vi "Execute Change Boolean Image Color.vi"(6 "Mouse Position":T1, 8 "User VI Ref":refnum<vi>, 9 "Menu Item Tag Suffix":string, 10 "Remaining Items":refnum<vi>[](array[refnum]), 11 "Affected Items":cluster{"Controls":refnum<vi>[]}) -> (0 "Fail transaction?":bool)   [LabVIEW 2021]
doc: "This VI will set a Boolean type that is input to the control's tag and stays persistent. It marks the data that is used in future application when changing themes.\n\n<b>Original</b>:This VI is part of a plug-in for modifying the LabVIEW shortcut menus. This is the execute VI which is called when the shortcut menu is chosen by the user. It performs the action of the selected menu item."
uses:
  Material-Scheme/Material-Scheme.lvclass
  <vilib>/Utility/miscctls.llb/LVPositionTypeDef.ctl
  Material SubVIs/Material SubVIs.lvlib
panel:
  # "All controls on this panel except \"Affected Items\" have been locked to prevent accidental edits. Changing the control names or types, other than the elements of the \"Affected Items\" cluster will make the VI unusable as a menu plugin.\n\nSee Context Help for each control for details about its use."
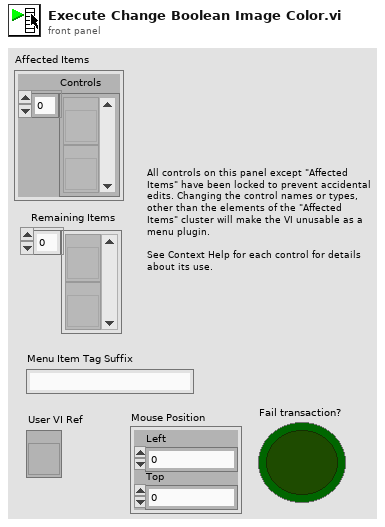
[diagram p1: front panel]
types:
  T1 = typedef "LVPositionTypeDef.ctl" = cluster{"Left":i32, "Top":i32}
  T2 = enum32{"invalid VI type", "Standard VI", "Control VI", "Global VI", "Polymorphic VI", "Configuration VI", "SubSystem", "Facade VI", "Method VI", "Statechart Diagram VI"}
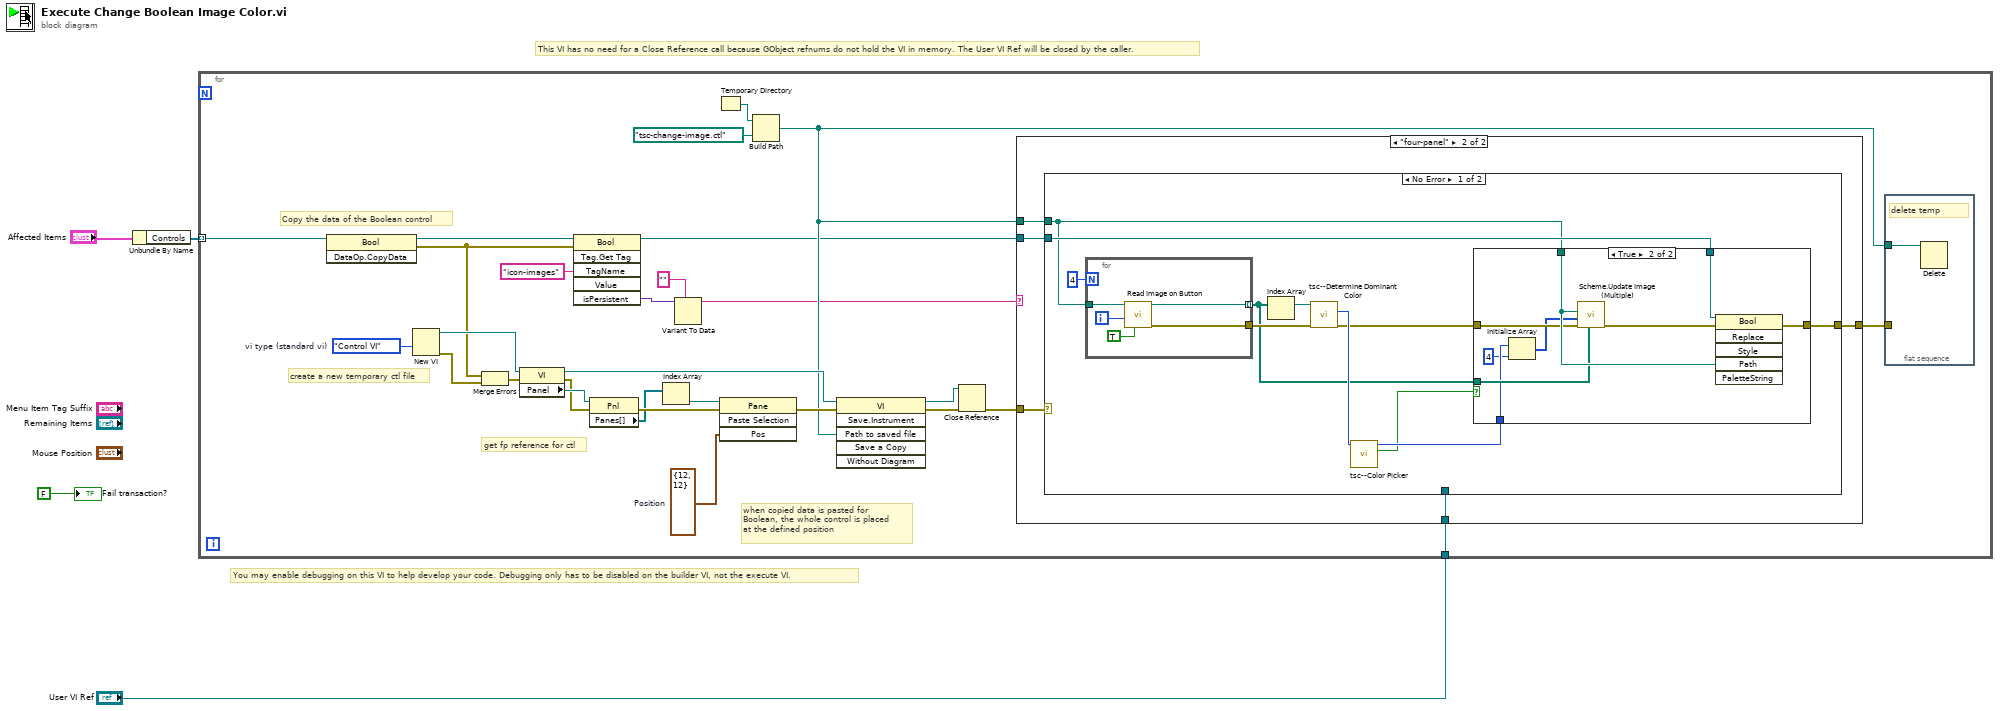
[diagram p0: block diagram]
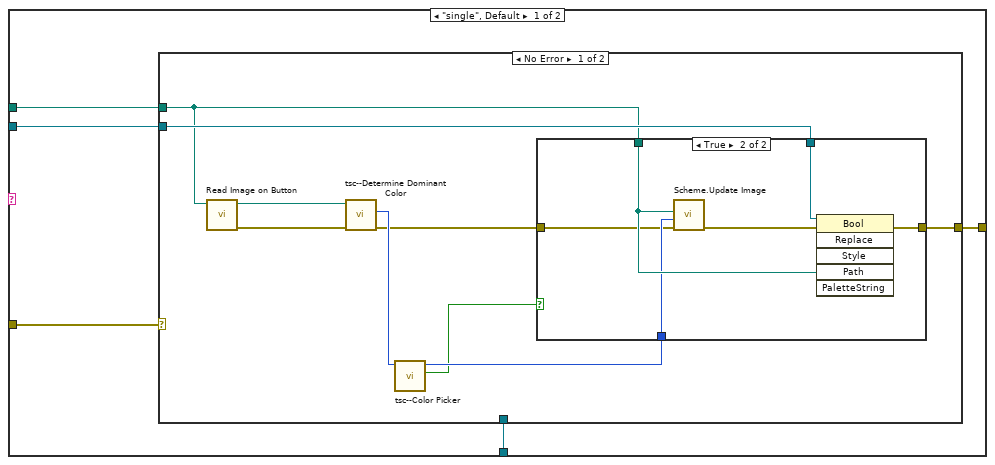
[diagram p2: hidden frame]
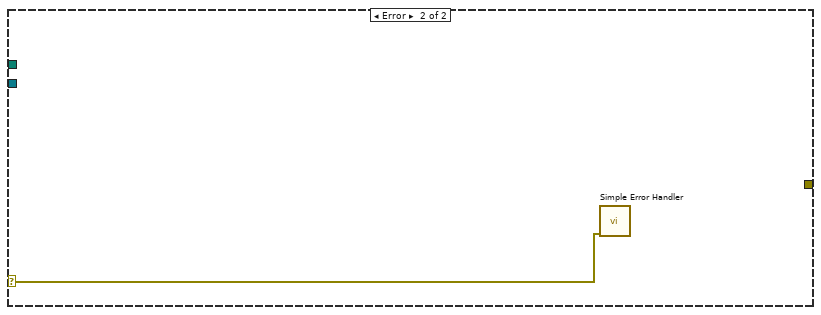
[diagram p4: hidden frame]
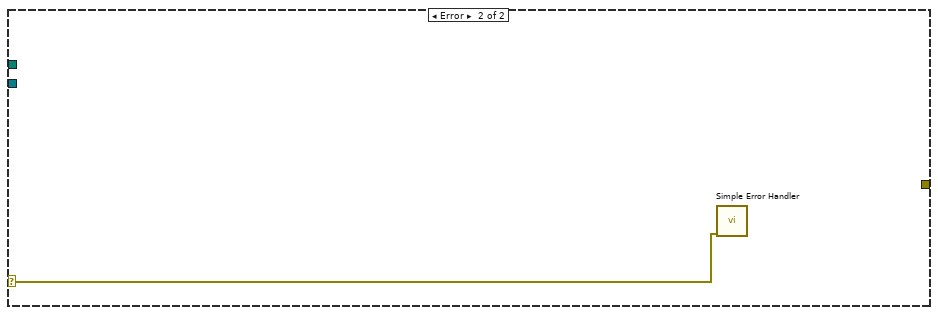
[diagram p6: hidden frame]
diagram:
  # "You may enable debugging on this VI to help develop your code. Debugging only has to be disabled on the builder VI, not the execute VI."
  # "This VI has no need for a Close Reference call because GObject refnums do not hold the VI in memory. The User VI Ref will be closed by the caller."
  n1 = Unbundle By Name("Affected Items") -> ("Controls"=w2:refnum<vi>[])
  n2 = for {
    tunnel: w2 -> [w24] mode=indexing
    tunnel: "User VI Ref" -> [w12]
    w21 = T2."Control VI"  # vi type (standard vi)
    w25 = T1 {"Left"=12, "Top"=12}  # Position
    # "when copied data is pasted for\nBoolean, the whole control is placed \nat the defined position"
    # "get fp reference for ctl"
    # "create a new temporary ctl file"
    # "Copy the data of the Boolean control"
    n3 = invoke class="Bool" method="DataOp.CopyData"(reference=w24) -> (reference out=w8:refnum<vi>, error out=w7:errorcluster)  [unwired: 2 in, 1 out]
    n4 = New VI(9:w21) -> (0:w19:errorcluster, 3:w20:refnum<vi>)  [unwired: 6 in]
    n5 = Merge Errors(w7, w19) -> (w23:errorcluster)
    n6 = property class="VI"(reference=w20, error in=w23) -> (reference out=w29:refnum<vi>, error out=w31:errorcluster, "Panel"=w32:refnum<vi>)
    n7 = invoke class="Bool" method="Tag.Get Tag"(reference=w8, error in=w7, "TagName"="icon-images" ("Tag Name")) -> (reference out=w6:refnum<vi>, "isPersistent"=w10:variant)  [unwired: 3 in, 4 out]
    n8 = property class="Pnl"(reference=w32, error in=w31) -> (error out=w28:errorcluster, "Panes[]"=w27:refnum<vi>[])  [unwired: 1 out]
    n9 = Index Array(array=w27) -> (element=w26:refnum<vi>)  [unwired: 1 in]
    n10 = Variant To Data(type="", Variant=w10) -> (data=w5:string)  [unwired: 1 in, 1 out]
    n11 = Temporary Directory() -> (w18:path)
    n12 = invoke class="Pane" method="Paste Selection"(reference=w26, error in=w28, "Pos"=w25) -> (error out=w30:errorcluster)  [unwired: 1 in, 3 out]
    n13 = Build Path(base path=w18, name or relative path=path "tsc-change-image.ctl") -> (appended path=w13:path)
    n14 = invoke class="VI" method="Save.Instrument"(reference=w29, error in=w30, "Path to saved file"=w13) -> (reference out=w15:refnum<vi>, error out=w22:errorcluster)  [unwired: 3 in, 4 out]
    n15 = Close Reference(reference=w15, error in (no error)=w22) -> (error out=w16:errorcluster)
    n16 = case shown="\"four-panel\"" w5 {
      tunnel: w16 -> [w37 w59]
      tunnel: [w36 w58] -> w14
      tunnel: w13 -> [w35 w57]
      tunnel: w12 -> [w34 w56]
      tunnel: w6 -> [w33 w55]
      frame "single", Default {
        n17 = case shown="No Error" w37 {
          selector: w37 -> [_ w54]
          tunnel: w35 -> [w44 _]
          tunnel: w33 -> [w46 _]
          tunnel: [w45 _] -> w36
          tunnel: w34 -> [_ _]
          frame No Error {
            n18 = call "Read Image on Button.vi"("File with Button"=w44) -> ("error out"=w42:errorcluster, "png file out"=w43:path)  [unwired: 9 in]
            n19 = call "tsc--Determine Dominant Color.vi"("error in"=w42, "orig file"=w43) -> ("error out"=w39:errorcluster, "maximum color"=w41:u32)  [unwired: 7 in, 1 out]
            n20 = call "tsc--Color Picker.vi"("input"=w41) -> ("accepted?"=w38:bool, "Resolved Color"=w40:u32)  [unwired: 9 in]
            n21 = case shown="True" w38 {
              tunnel: w46 -> [_ w52]
              tunnel: [w47 w51] -> w45
              tunnel: w44 -> [_ w50]
              tunnel: w40 -> [_ w49]
              tunnel: w39 -> [w47 w48]
              frame False {
              }
              frame True {
                n22 = call "Scheme.Update Image.vi"("error in"=w48, "New Color"=w49, "New Control"=w50) -> ("error out"=w53:errorcluster)  [unwired: 7 in, 1 out]
                n23 = invoke class="Bool" method="Replace"(reference=w52, error in=w53, "Path"=w50) -> (error out=w51:errorcluster)  [unwired: 3 in, 5 out]
              }
            }
          }
          frame Error {
            n24 = call <vilib>:"Simple Error Handler.vi"("error in (no error)"=w54) -> ()  [unwired: 4 in, 5 out]
          }
        }
      }
      frame "four-panel" {
        n25 = case shown="No Error" w59 {
          selector: w59 -> [_ w86]
          tunnel: w57 -> [w68 _]
          tunnel: w55 -> [w70 _]
          tunnel: [w69 _] -> w58
          tunnel: w56 -> [_ _]
          frame No Error {
            n26 = for {
              N: 4 -> [_]
              tunnel: [w74] -> w67
              tunnel: w68 -> [w75]
              tunnel: [w72] -> w60 mode=indexing
              i -> [w73]
              n27 = call "Read Image on Button.vi"("Append Name?"=TRUE, "image item"=w73, "File with Button"=w75) -> ("error out"=w74:errorcluster, "png file out"=w72:path)  [unwired: 7 in]
            }
            n28 = Index Array(array=w60) -> (element=w61:path)  [unwired: 1 in]
            n29 = call "tsc--Determine Dominant Color.vi"("error in"=w67, "orig file"=w61) -> ("error out"=w64:errorcluster, "maximum color"=w66:u32)  [unwired: 7 in, 1 out]
            n30 = call "tsc--Color Picker.vi"("input"=w66) -> ("accepted?"=w63:bool, "Resolved Color"=w65:u32)  [unwired: 9 in]
            n31 = case shown="True" w63 {
              tunnel: w70 -> [_ w84]
              tunnel: [w76 w83] -> w69
              tunnel: w68 -> [_ w82]
              tunnel: w65 -> [_ w79]
              tunnel: w64 -> [w76 w81]
              tunnel: w60 -> [_ w80]
              frame False {
              }
              frame True {
                n32 = Initialize Array(w79, 4 ("dimension size")) -> (w77:u32[])
                n33 = call "Scheme.Update Image (Multiple).vi"("Replace Image"=w80, "error in"=w81, "New Color"=w77, "New Control"=w82) -> ("error out"=w85:errorcluster)  [unwired: 5 in, 2 out]
                n34 = invoke class="Bool" method="Replace"(reference=w84, error in=w85, "Path"=w82) -> (error out=w83:errorcluster)  [unwired: 3 in, 5 out]
              }
            }
          }
          frame Error {
            n35 = call <vilib>:"Simple Error Handler.vi"("error in (no error)"=w86) -> ()  [unwired: 4 in, 5 out]
          }
        }
      }
    }
    n36 = flat-sequence {
      tunnel: w14 -> [_]
      tunnel: w13 -> [w87]
      frame #0 {
        # "delete temp"
        n37 = Delete(path (use dialog)=w87) -> ()  [unwired: 4 in, 3 out]
      }
    }
  }
  "Fail transaction?" <- FALSE ("Fail transaction?")
